vi "Actor Core.vi"(8 "error in":errorcluster, 11 "Data Manager in":refnum<class "Data Manager.lvclass">) -> (0 "error out":errorcluster, 3 "Actor out":refnum<class "Actor.lvclass">)   [LabVIEW 2017, in "2. Basic Panel Actors.lvlib" / "Data Manager.lvclass"]
doc: "The user interface for this panel.\n----\nCopyright: MGI 2016\nAuthor: Derek Trepanier"
uses:
  Data Manager.lvclass
  panel-actors/Source/Panel Actor/Panel Actor.lvclass
  <vilib>/measure/NI_MABase.lvlib
  Data Viewer/Data Viewer.lvclass
  panel-manager/Source/MGI-Panel Manager.lvlib
  panel-manager/Source/Panel/Window/Window.vi
  panel-manager/Source/Panel/Window/Window.lvclass
  panel-manager/Source/Window Position/Reference Position/Ref Display/Ref Display.vi
  panel-manager/Source/Window Position/Reference Position/Ref Display/Ref Display.lvclass
  panel-manager/Source/Window Position/Reference Position/Size/Reference Size/Reference Size.vi
  panel-manager/Source/Window Position/Reference Position/Size/Reference Size/Reference Size.lvclass
  panel-manager/Source/Window Position/Reference Position/Offset/Cascade/Cascade.lvclass
  D:/test/LabView_PanelManager/panel-actors/Source/Panel Actor/Panel Actor.lvclass
  D:/test/LabView_PanelManager/panel-manager/Source/Window Position/Reference Position/Offset/Offset.lvclass
  D:/test/LabView_PanelManager/panel-manager/Source/Window Position/Reference Position/Size/Size.lvclass
  D:/test/LabView_PanelManager/panel-manager/Source/Window Position/Reference Position/Reference Position.lvclass
  D:/test/LabView_PanelManager/panel-manager/Source/Window Position/Window Position.lvclass
  D:/test/LabView_PanelManager/panel-manager/Source/Panel/Panel.lvclass
  <vilib>/ActorFramework/Actor/Actor.lvclass
panel:
  in  "View in New Window":bool
  in  "Datasets":i32[](listbox)
  in  "New Data Set":bool
  # "Drag dataset(s) from me"
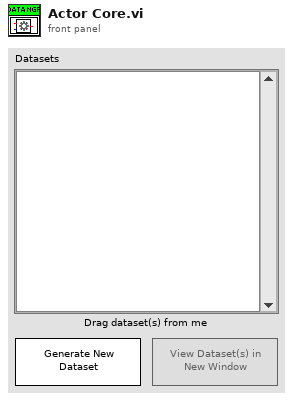
[diagram p1: front panel]
types:
  T1 = enum8{"Enabled", "Disabled", "Disabled and Grayed Out"}
  T2 = enum16{"Sine Wave", "Triangle Wave", "Square Wave", "Sawtooth Wave"}
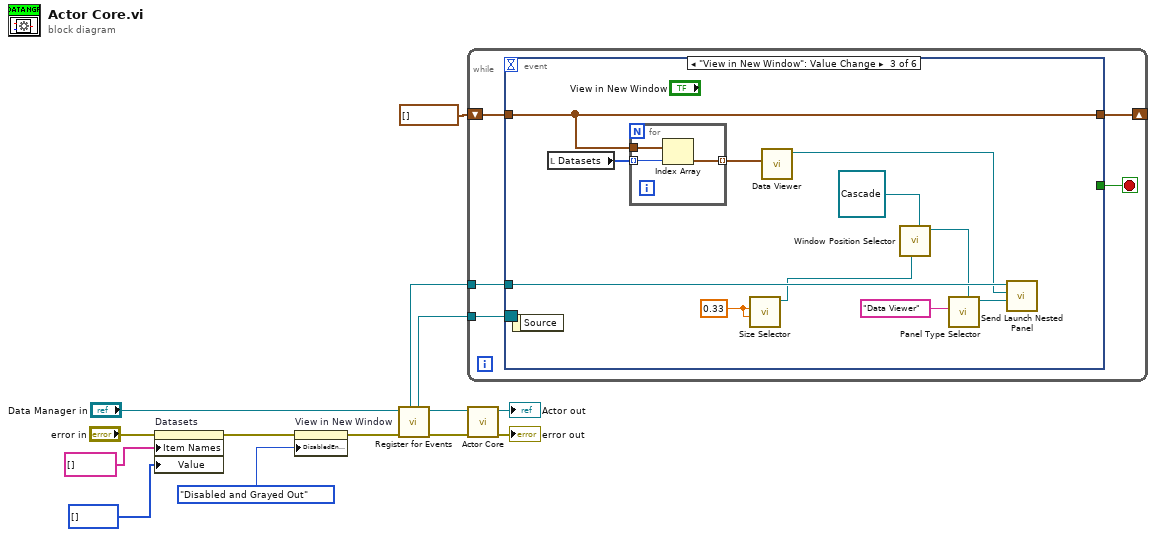
[diagram p0: block diagram]
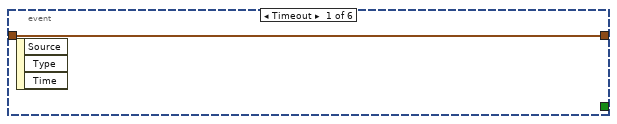
[diagram p2: hidden frame]
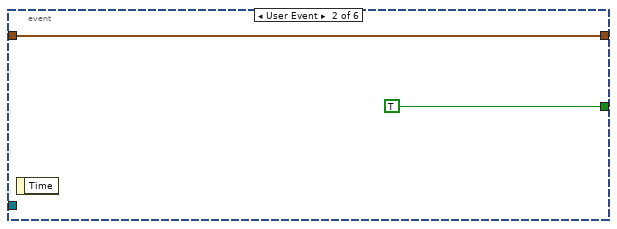
[diagram p3: hidden frame]
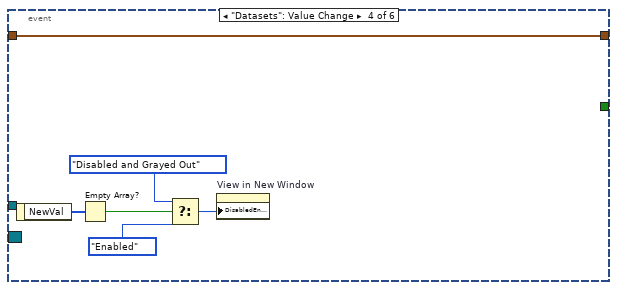
[diagram p4: hidden frame]
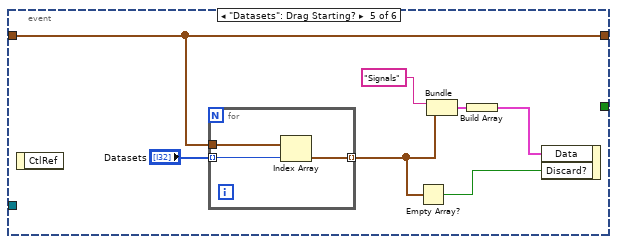
[diagram p5: hidden frame]
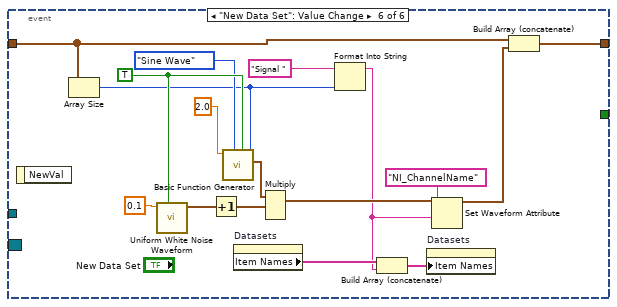
[diagram p6: hidden frame]
diagram:
  n1 = property on="Datasets" class="LstBox (strict)"(error in="error in", "Item Names"=string[] [], "Value"=i32[] [] ("Value (Signaling)")) -> (error out=w5:errorcluster)  [unwired: 1 in, 1 out]
  n2 = property on="View in New Window" class="Bool"(error in=w5, "DisabledEnum"=T1."Disabled and Grayed Out" ("Disabled")) -> (error out=w4:errorcluster)  [unwired: 1 in, 1 out]
  n3 = call "Register for Events.vi"("Error In"=w4, "Panel Actor in"="Data Manager in") -> ("Error Out"=w1:errorcluster, "Panel Actor out"=w8:refnum<class "Data Manager.lvclass">, "Pnl Actor"=w7:refnum<event-registration>, "Self Enqueuer"=w6:refnum<class "Message Enqueuer.lvclass">)  [unwired: 5 in, 1 out]
  n4 = while {
    tunnel: w7 -> [w19]
    tunnel: w6 -> [w18]
    shift-right: [w16] -> _
    shift-left: waveform(dbl)[] [] -> [w15]
    stop <- w17 stop-if-true
    n5 = event shown="[2] \"View in New Window\": Value Change" {
      selector: w19 -> [_ _ _ _ _ _]
      dyn-events: _ -> [_ _ _ _ _ _]
      timeout: _ -> [_ _ _ _ _ _]
      tunnel: w18 -> [_ _ w30 _ _ _]
      tunnel: [_ TRUE _ _ _ _] -> w17
      tunnel: [w20 w21 w33 w37 w48 w61] -> w16
      tunnel: w15 -> [w20 w21 w33 w37 w48 w60]
      event Timeout {
        n6 = event-data() -> ()  [unwired: 1 in, 3 out]
      }
      event User Event {
        n7 = event-data() -> ()  [unwired: 1 in, 1 out]
      }
      event "View in New Window": Value Change {
        w24 = 0.33 ("Width Scale")
        n8 = event-data() -> ()  [unwired: 1 in, 1 out]
        n9 = local read "Datasets"() -> (w32:i32[])
        n10 = for {
          tunnel: w33 -> [w36]
          tunnel: w32 -> [w35] mode=indexing
          tunnel: [w34] -> w31 mode=indexing
          n11 = Index Array(array=w36, index=w35) -> (element=w34:waveform(dbl))
        }
        n12 = call-poly "Size Selector.vi"("Height Scale"=w24, "Width Scale"=w24) -> ("Static Out"=w25:refnum<class "Reference Size.lvclass">)  [unwired: 8 in, 1 out]
        n13 = call "Data Viewer.vi"("Starting Waveforms"=w31) -> ("Data Viewer out"=w23:refnum<class "Data Viewer.lvclass">)  [unwired: 9 in, 1 out]
        n14 = call-poly "Window Position Selector.vi"("Offset"=refnum<class "Cascade.lvclass"> refnum ("MGI-Panel Manager.lvlib:Cascade.lvclass"), "Size"=w25) -> ("Ref Display out"=w27:refnum<class "Ref Display.lvclass">)  [unwired: 8 in, 1 out]
        n15 = call-poly "Panel Type Selector.vi"("Window Position"=w27, "Default Title"="Data Viewer") -> ("Window out"=w29:refnum<class "Window.lvclass">)  [unwired: 8 in, 1 out]
        n16 = call "Send Launch Nested Panel.vi"("Panel"=w29, "Nested Panel Actor"=w23, "Self Enqueuer in"=w30) -> ()  [unwired: 6 in, 3 out]
      }
      event "Datasets": Value Change {
        n17 = event-data() -> ("NewVal"=w42:i32[])  [unwired: 1 in]
        n18 = Empty Array?(array=w42) -> (empty?=w41:bool)
        n19 = Select(t=T1."Disabled and Grayed Out" ("Disabled"), s=w41, f=T1."Enabled" ("Disabled")) -> (s? t:f=w40:T1)
        n20 = property on="View in New Window" class="Bool"("DisabledEnum"=w40) -> ()  [unwired: 2 in, 2 out]
      }
      event "Datasets": Drag Starting? {
        n21 = event-data() -> ()  [unwired: 1 in, 1 out]
        n22 = for {
          tunnel: "Datasets" -> [w51] mode=indexing
          tunnel: w48 -> [w52]
          tunnel: [w50] -> w44 mode=indexing
          n23 = Index Array(array=w52, index=w51) -> (element=w50:waveform(dbl))
        }
        n24 = Empty Array?(array=w44) -> (empty?=w43:bool)
        n25 = Bundle("Signals", w44) -> (w46:cluster{string, waveform(dbl)[]})  [unwired: 1 in]
        n26 = Build Array(w46) -> (w45:cluster{string, waveform(dbl)[]}[])
        n27 = event-data("Data"=w45, "Discard?"=w43) -> ()  [unwired: 1 in, 1 out]
      }
      event "New Data Set": Value Change {
        w64 = TRUE ("reset signal")
        n28 = event-data() -> ()  [unwired: 1 in, 1 out]
        n29 = Array Size(array=w60) -> (size(s)=w59:i32)
        n30 = call <vilib>:"Uniform White Noise Waveform.vi"("reset signal"=w64, "amplitude"=0.1) -> ("signal out"=w67:waveform(dbl))  [unwired: 8 in, 1 out]
        n31 = Increment(x=w67) -> (x+1=w66:waveform(dbl))
        n32 = call <vilib>:"Basic Function Generator.vi"("offset"=w59, "reset signal"=w64, "signal type"=T2."Sine Wave", "frequency"=2.0) -> ("signal out"=w65:waveform(dbl))  [unwired: 5 in, 2 out]
        n33 = property on="Datasets" class="LstBox (strict)"() -> ("Item Names"=w57:string[])  [unwired: 2 in, 2 out]
        n34 = Multiply(1:w66, 2:w65) -> (0:w62:waveform(dbl))  [unwired: 1 in, 1 out]
        n35 = Format Into String(initial string="Signal ", w59) -> (resulting string=w54:string)  [unwired: 2 in, 1 out]
        n36 = Build Array (concatenate)(w57, w54) -> (w56:string[])
        n37 = property on="Datasets" class="LstBox (strict)"("Item Names"=w56) -> ()  [unwired: 2 in, 2 out]
        n38 = Set Waveform Attribute(5:w54, 6:"NI_ChannelName" ("name"), 7:w62) -> (3:w55:waveform(dbl))  [unwired: 1 in, 2 out]
        n39 = Build Array (concatenate)(w60, w55) -> (w61:waveform(dbl)[])
      }
    }
  }
  n40 = call-parent "Actor Core.vi"("error in"=w1, "Panel Actor in"=w8) -> ("error out"=→"error out":errorcluster, "Actor out"=→"Actor out":refnum<class "Actor.lvclass">)  [unwired: 8 in]
